vi "insertReturnTrip.vi"(3 "Galvo Array in":dbl[][](array[numeric])=array2x5000[10000 elements], 4 "Camera in":refnum<class "Camera.lvclass">, 5 "Galvo obj array":refnum<class "Galvonometer.lvclass">[](array[class])=[refnum, refnum], 6 "Scan in":refnum<class "Scan.lvclass">) -> (0 "Galvo array out":dbl[][](array[numeric]), 1 "inactive A-scans":dbl=130.0, 2 "Delay A":dbl)   [LabVIEW 2017]
uses:
  classes/Scans/Scan.lvclass
  classes/HardwareObjects/Camera/Camera.lvclass
  classes/HardwareObjects/Galvonometer/Galvonometer.lvclass
  classes/Scans/Scan.lvclass/Scan.ctl
  classes/HardwareObjects/Camera/Camera.lvclass/Camera.ctl
  classes/HardwareObjects/Galvonometer/Galvonometer.lvclass/Galvonometer.ctl
  <vilib>/Analysis/1siggen.llb/Ramp Pattern by Samples.vi
  classes/HardwareObjects/Camera/Read Max Frequency (kHz).vi
  classes/HardwareObjects/Galvonometer/Read Output Scale Factor (V_degrees).vi
  classes/HardwareObjects/Galvonometer/Read Max Scan Angle (degrees).vi
  classes/Scans/Read Total B-Scans.vi
  classes/Scans/Read A scans.vi
  classes/Scans/Read Bidirectional.vi
  <vilib>/Analysis/NI_AALBase.lvlib
panel:
  out "irt tic":dbl format="%_19f"
  out "x-y":dbl
  out "irt toc":dbl format="%_19f"
  in  "debug":bool
  out "XY Graph":cluster{"Ramp Pattern":dbl[], dbl[]}[](graph)
  out "Return time (s)":dbl=1.1451474377326093e-06
  out "Return distance (°)":dbl=0.005010020040080165
  out "Max angular velocity (°/s)":i32=8750
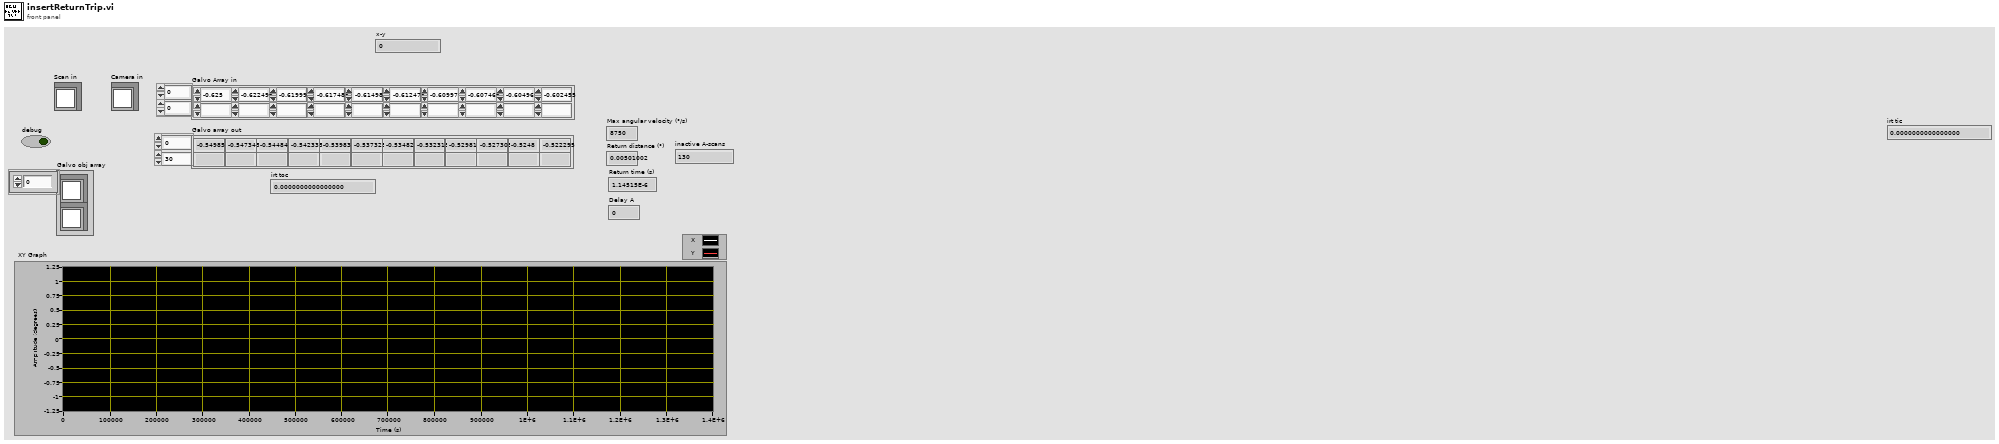
[diagram p1: front panel]
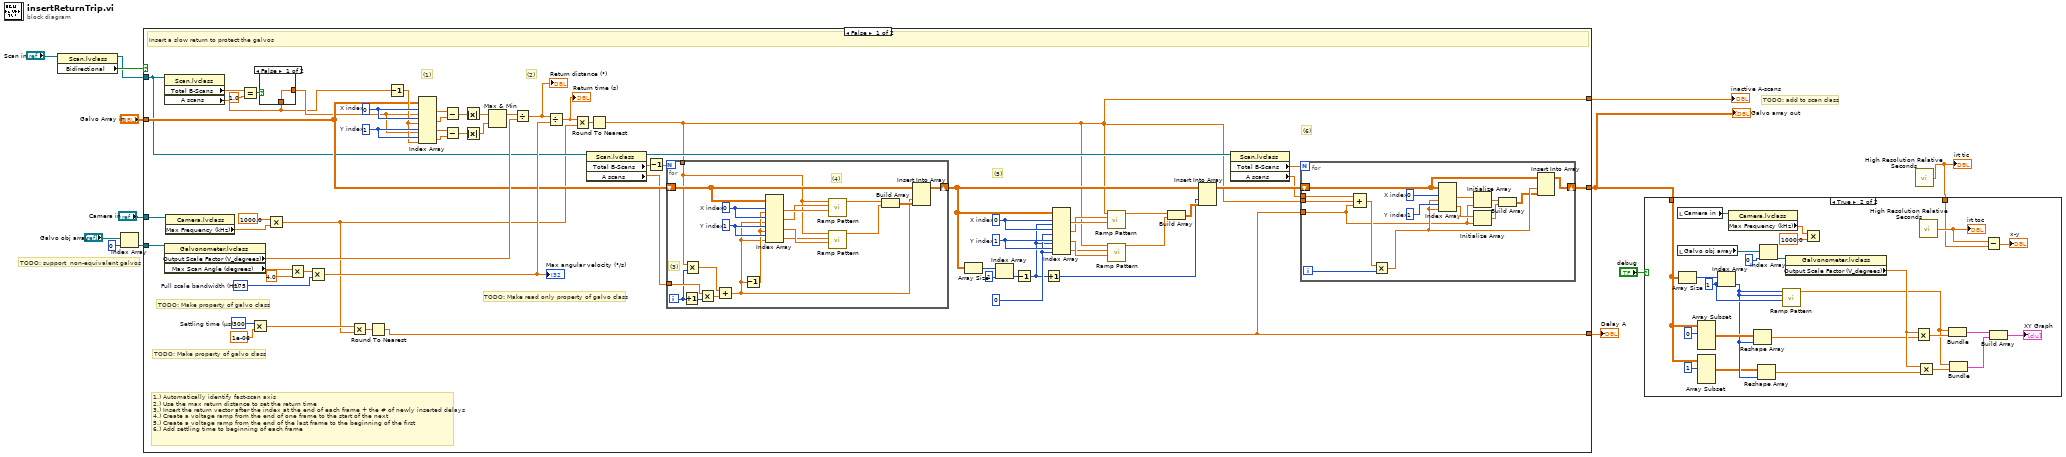
[diagram p0: block diagram]
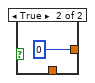
[diagram p2: hidden frame]
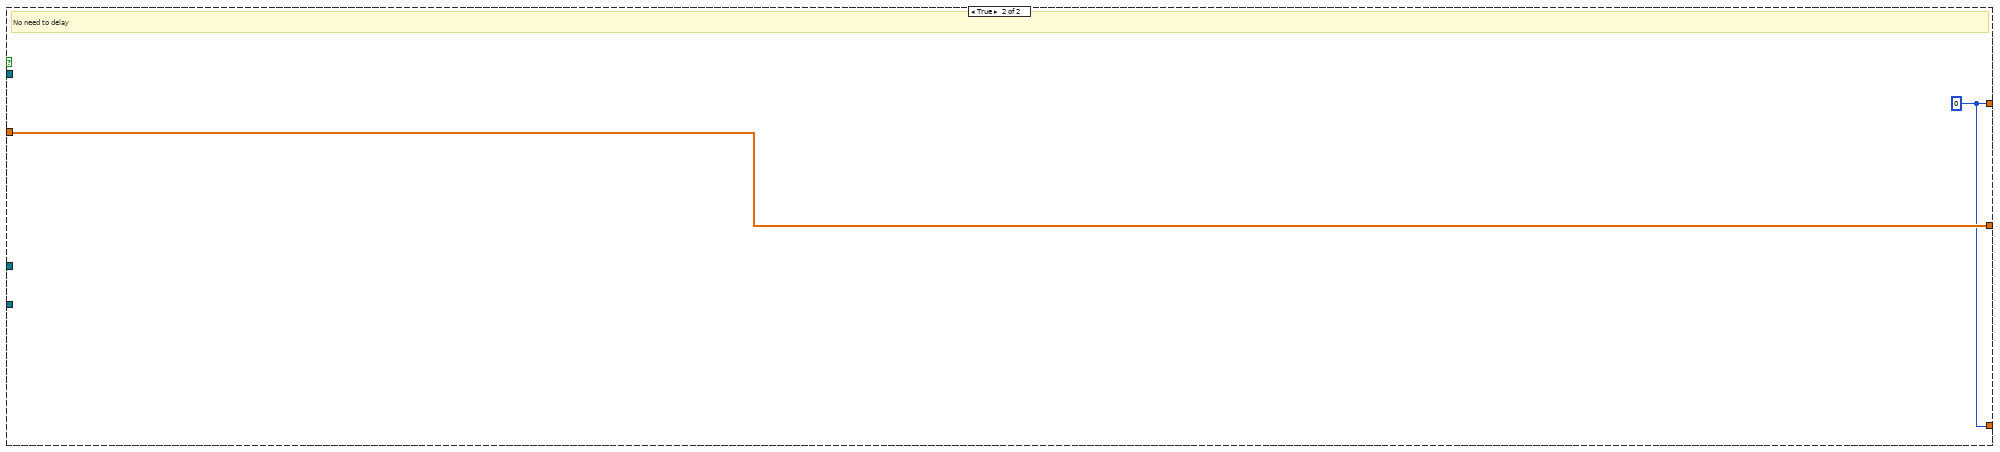
[diagram p3: hidden frame]
diagram:
  # "TODO: add to scan class"
  # "TODO: support  non-equivalent galvos"
  n1 = property class="Scan.lvclass"(reference="Scan in") -> (reference out=w11:refnum<class "Scan.lvclass">, "Bidirectional"=w12:bool)  [unwired: 1 in, 1 out]
  n2 = Index Array(array="Galvo obj array", index=0) -> (element=w4:refnum<class "Galvonometer.lvclass">)
  n3 = case shown="False" w12 {
    tunnel: "Galvo Array in" -> [w57 w114]
    tunnel: [w18 w114] -> w9
    tunnel: w11 -> [w33 _]
    tunnel: w4 -> [w67 _]
    tunnel: "Camera in" -> [w66 _]
    tunnel: [w17 w113] -> w3
    tunnel: [w14 w113] -> w2
    frame False {
      w25 = 300  # Settling time (µs)
      w47 = 0
      w49 = 1  # Y index
      w48 = 0  # X index
      w15 = 175  # Full scale bandwidth (Hz)
      w75 = 1  # Y index
      w76 = 0  # X index
      # "(6)"
      # "TODO: Make property of galvo class"
      # "(5)"
      # "(2)"
      # "(1)"
      # "1.) Automatically identify fast-scan axis\n2.) Use the max return distance to set the return time \n3.) Insert the return vector after the index at the end of each frame + the # of newly inserted delays\n4.) Create a voltage ramp from the end of one frame to the start of the next\n5.) Create a voltage ramp from the end of the last frame to the beginning of the first\n6.) Add settling time to beginning of each frame"
      # "TODO: Make read only property of galvo class"
      # "TODO: Make property of galvo class"
      # "Insert a slow return to protect the galvos"
      n4 = property class="Galvonometer.lvclass"(reference=w67) -> ("Output Scale Factor (V_degrees)"=w62:dbl, "Max Scan Angle (degrees)"=w61:dbl)  [unwired: 1 in, 2 out]
      n5 = property class="Scan.lvclass"(reference=w33) -> ("Total B-Scans"=w32:dbl, "A scans"=w28:dbl)  [unwired: 1 in, 2 out]
      n6 = property class="Camera.lvclass"(reference=w66) -> ("Max Frequency (kHz)"=w53:sgl)  [unwired: 1 in, 2 out]
      n7 = Equal?(x=w32, y=1.0) -> (x = y?=w30:bool)
      n8 = Multiply(x=w25, y=1e-06) -> (x*y=w24:dbl)
      n9 = case shown="False" w30 {
        tunnel: [w92 0] -> w29
        tunnel: w28 -> [w92 _]
        frame False {
          # "Compare end to start of next"
        }
        frame True {
          # "Compare end to beginning"
        }
      }
      n10 = Multiply(x=1000.0 ("y"), y=w53) -> (x*y=w23:dbl)
      n11 = Multiply(x=w61, y=4.0) -> (x*y=w60:dbl)
      n12 = Multiply(x=w60, y=w15) -> (x*y=w58:dbl)
      "Max angular velocity (°/s)" <- w58
      n13 = Multiply(x=w24, y=w23) -> (x*y=w22:dbl)
      n14 = Round To Nearest(number=w22) -> (nearest integer value=w14:dbl)
      n15 = Decrement(x=w28) -> (x-1=w74:dbl)
      n16 = Index Array(array=w57, index (row) #1=w76, index (col) #1=w29, index (row) #2=w76, index (col) #2=w74, index (row) #3=w75, index (col) #3=w29, index (row) #4=w75, index (col) #4=w74) -> (element #1=w73:dbl, element #2=w72:dbl, element #3=w71:dbl, element #4=w70:dbl)
      n17 = Subtract(x=w73, y=w72) -> (x-y=w69:dbl)
      n18 = Subtract(x=w71, y=w70) -> (x-y=w68:dbl)
      n19 = Absolute Value(x=w69) -> (abs(x)=w65:dbl)
      n20 = Absolute Value(x=w68) -> (abs(x)=w64:dbl)
      n21 = Max & Min(x=w65, y=w64) -> (max(x,y)=w63:dbl)  [unwired: 1 out]
      n22 = Divide(x=w63, y=w62) -> (x/y=w59:dbl)
      "Return distance (°)" <- w59
      n23 = Divide(x=w59, y=w58) -> (x/y=w55:dbl)
      "Return time (s)" <- w55
      n24 = Multiply(x=w55, y=w23) -> (x*y=w52:dbl)
      n25 = property class="Scan.lvclass"(reference=w33) -> (reference out=w21:refnum<class "Scan.lvclass">, "Total B-Scans"=w51:dbl, "A scans"=w56:dbl)  [unwired: 1 in, 1 out]
      n26 = Round To Nearest(number=w52) -> (nearest integer value=w17:dbl)
      n27 = Decrement(x=w51) -> (x-1=w50:dbl)
      n28 = for {
        N: w50 -> [_]
        shift-right: [w110] -> w38
        shift-left: w57 -> [w104]
        tunnel: w56 -> [w111]
        tunnel: w17 -> [w99]
        i -> [w106]
        w103 = 1  # Y index
        w102 = 0  # X index
        # "(4)"
        # "(3)"
        n29 = Increment(x=w106) -> (x+1=w112:i32)
        n30 = Multiply(x=w99, y=w106) -> (x*y=w105:dbl)
        n31 = Multiply(x=w111, y=w112) -> (x*y=w107:dbl)
        n32 = Add(x=w105, y=w107) -> (x+y=w94:dbl)
        n33 = Decrement(x=w94) -> (x-1=w95:dbl)
        n34 = Index Array(array=w104, index (row) #1=w102, index (col) #1=w95, index (row) #2=w102, index (col) #2=w94, index (row) #3=w103, index (col) #3=w95, index (row) #4=w103, index (col) #4=w94) -> (element #1=w101:dbl, element #2=w100:dbl, element #3=w98:dbl, element #4=w97:dbl)
        n35 = call-poly <vilib>:"Ramp Pattern.vi"("start"=w101, "end"=w100, "samples"=w99) -> ("Ramp Pattern"=w109:dbl[])  [unwired: 7 in, 1 out]
        n36 = call-poly <vilib>:"Ramp Pattern.vi"("start"=w98, "end"=w97, "samples"=w99) -> ("Ramp Pattern"=w108:dbl[])  [unwired: 7 in, 1 out]
        n37 = Build Array(w109, w108) -> (w96:dbl[][])
        n38 = Insert Into Array(array=w104, index (col)=w94, new element=w96) -> (w110:dbl[][])  [unwired: 1 in]
      }
      n39 = Array Size(array=w38) -> (size(s)=w46:i32[])
      n40 = Index Array(array=w46, index=1) -> (element=w36:i32)
      n41 = Decrement(x=w36) -> (x-1=w35:i32)
      n42 = Increment(x=w35) -> (x+1=w34:i32)
      n43 = Index Array(array=w38, index (row) #1=w48, index (col) #1=w35, index (row) #2=w48, index (col) #2=w47, index (row) #3=w49, index (col) #3=w35, index (row) #4=w49, index (col) #4=w47) -> (element #1=w44:dbl, element #2=w43:dbl, element #3=w42:dbl, element #4=w41:dbl)
      n44 = call-poly <vilib>:"Ramp Pattern.vi"("start"=w44, "end"=w43, "samples"=w17) -> ("Ramp Pattern"=w40:dbl[])  [unwired: 7 in, 1 out]
      n45 = call-poly <vilib>:"Ramp Pattern.vi"("start"=w42, "end"=w41, "samples"=w17) -> ("Ramp Pattern"=w39:dbl[])  [unwired: 7 in, 1 out]
      n46 = Build Array(w40, w39) -> (w37:dbl[][])
      n47 = Insert Into Array(array=w38, index (col)=w34, new element=w37) -> (w19:dbl[][])  [unwired: 1 in]
      n48 = property class="Scan.lvclass"(reference=w21) -> ("Total B-Scans"=w20:dbl, "A scans"=w16:dbl)  [unwired: 1 in, 2 out]
      n49 = for {
        N: w20 -> [_]
        shift-right: [w78] -> w18
        shift-left: w19 -> [w81]
        tunnel: w17 -> [w89]
        tunnel: w16 -> [w88]
        tunnel: w14 -> [w77]
        i -> [w90]
        w86 = 1  # Y index
        w91 = 0  # X index
        n50 = Compound Arithmetic op=unknown(w88, w89, w77) -> (w87:dbl)
        n51 = Multiply(x=w87, y=w90) -> (x*y=w80:dbl)
        n52 = Index Array(array=w81, index (row) #1=w91, index (col) #1=w80, index (row) #2=w86, index (col) #2=w80) -> (element #1=w85:dbl, element #2=w84:dbl)
        n53 = Initialize Array(w85, w77) -> (w83:dbl[])
        n54 = Initialize Array(w84, w77) -> (w82:dbl[])
        n55 = Build Array(w83, w82) -> (w79:dbl[][])
        n56 = Insert Into Array(array=w81, index (col)=w80, new element=w79) -> (w78:dbl[][])  [unwired: 1 in]
      }
    }
    frame True {
      w113 = 0
      # "No need to delay"
    }
  }
  "Galvo array out" <- w9
  "inactive A-scans" <- w3
  "Delay A" <- w2
  n57 = call <vilib>:"High Resolution Relative Seconds.vi"() -> ("relative seconds"=w1:dbl)
  "irt tic" <- w1
  n58 = case shown="True" "debug" {
    tunnel: w9 -> [_ w138]
    tunnel: w1 -> [_ w115]
    frame False {
    }
    frame True {
      w136 = 1 ("index")
      n59 = local read "Camera in"() -> (w121:refnum<class "Camera.lvclass">)
      n60 = local read "Galvo obj array"() -> (w129:refnum<class "Galvonometer.lvclass">[])
      n61 = Array Size(array=w138) -> (size(s)=w137:i32[])
      n62 = Array Subset(array=w138, index (row)=0 ("index")) -> (w133:dbl[][])  [unwired: 3 in]
      n63 = Array Subset(array=w138, index (row)=1 ("index")) -> (w131:dbl[][])  [unwired: 3 in]
      n64 = Index Array(array=w137, index=w136) -> (element=w132:i32)
      n65 = property class="Camera.lvclass"(reference=w121) -> ("Max Frequency (kHz)"=w119:sgl)  [unwired: 1 in, 2 out]
      n66 = Reshape Array(w133, w132) -> (w124:dbl[])
      n67 = Reshape Array(w131, w132) -> (w125:dbl[])
      n68 = Index Array(array=w129, index=0) -> (element=w127:refnum<class "Galvonometer.lvclass">)
      n69 = call-poly <vilib>:"Ramp Pattern.vi"("start"=w136, "end"=w132, "samples"=w132) -> ("Ramp Pattern"=w120:dbl[])  [unwired: 7 in, 1 out]
      n70 = property class="Galvonometer.lvclass"(reference=w127) -> ("Output Scale Factor (V_degrees)"=w126:dbl)  [unwired: 1 in, 2 out]
      n71 = Multiply(x=w119, y=sgl 1000.0) -> ()  [unwired: 1 out]
      n72 = Multiply(x=w126, y=w124) -> (x*y=w123:dbl[])
      n73 = Multiply(x=w126, y=w125) -> (x*y=w122:dbl[])
      n74 = call <vilib>:"High Resolution Relative Seconds.vi"() -> ("relative seconds"=w116:dbl)
      "irt toc" <- w116
      n75 = Bundle("Ramp Pattern"=w120, w123) -> (w135:cluster{"Ramp Pattern":dbl[], dbl[]})  [unwired: 1 in]
      n76 = Bundle("Ramp Pattern"=w120, w122) -> (w134:cluster{"Ramp Pattern":dbl[], dbl[]})  [unwired: 1 in]
      n77 = Subtract(x=w116, y=w115) -> (x-y=→"x-y":dbl)
      n78 = Build Array(w135, w134) -> (→"XY Graph":cluster{"Ramp Pattern":dbl[], dbl[]}[])
    }
  }
